vi "d7seg.vi"(0 "Numeric":dbl min=0.0 max=9.0 step=1.0) -> (20 "a":bool, 21 "b":bool, 22 "c":bool, 23 "d":bool, 24 "e":bool, 25 "f":bool, 26 "g":bool, 27 "h":bool)   [LabVIEW 2022 SP3]
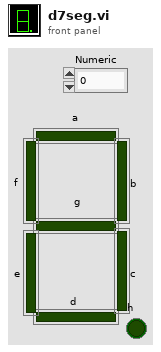
[diagram p1: front panel]
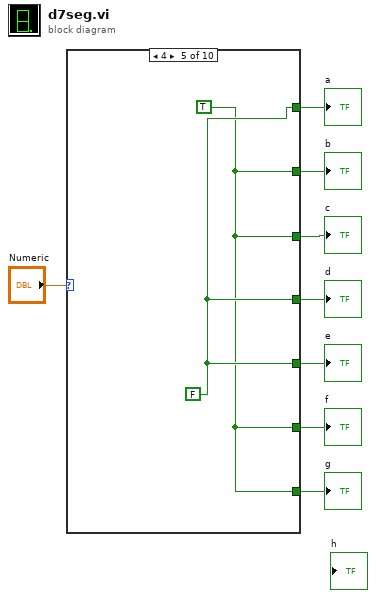
[diagram p0: block diagram]
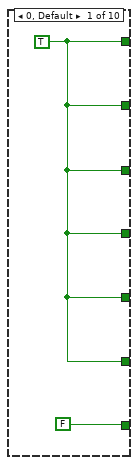
[diagram p2: hidden frame]
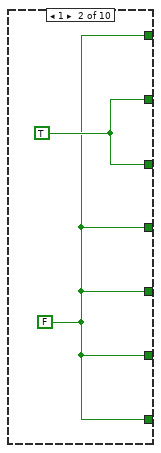
[diagram p3: hidden frame]
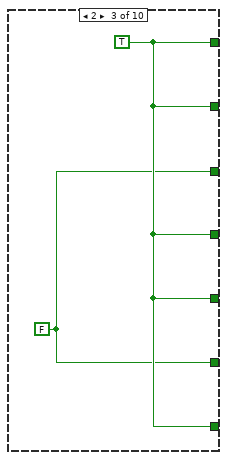
[diagram p4: hidden frame]
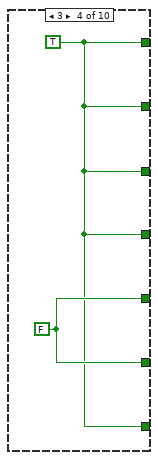
[diagram p5: hidden frame]
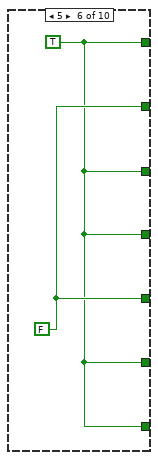
[diagram p6: hidden frame]
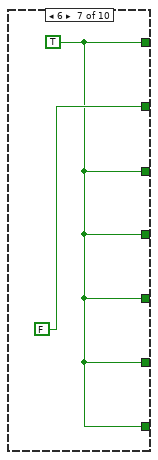
[diagram p7: hidden frame]
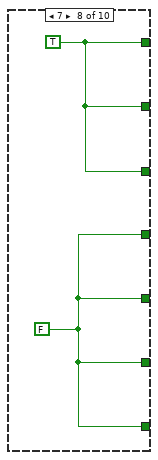
[diagram p8: hidden frame]
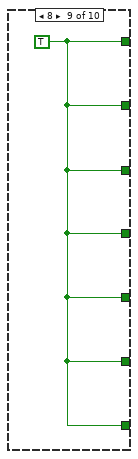
[diagram p9: hidden frame]
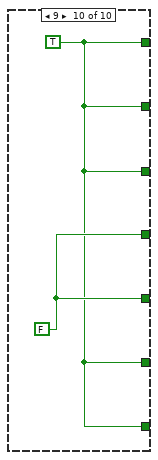
[diagram p10: hidden frame]
diagram:
  n1 = case shown="4" "Numeric" {
    tunnel: [w10 w11 w14 w15 w18 w19 w21 w24 w25 w26] -> w7
    tunnel: [w10 w12 w14 w15 w17 w20 FALSE w24 w25 w26] -> w6
    tunnel: [w10 w12 w13 w15 w17 w19 w21 w24 w25 w26] -> w5
    tunnel: [w10 w11 w14 w15 w18 w19 w21 w23 w25 w27] -> w4
    tunnel: [w10 w11 w14 w16 w18 w20 w21 w23 w25 w27] -> w3
    tunnel: [w10 w11 w13 w16 w17 w19 w21 w23 w25 w26] -> w2
    tunnel: [FALSE w11 w14 w15 w17 w19 w21 w23 w25 w26] -> w1
    frame 0, Default {
      w10 = TRUE
    }
    frame 1 {
      w11 = FALSE
      w12 = TRUE
    }
    frame 2 {
      w13 = FALSE
      w14 = TRUE
    }
    frame 3 {
      w16 = FALSE
      w15 = TRUE
    }
    frame 4 {
      w18 = FALSE
      w17 = TRUE
    }
    frame 5 {
      w20 = FALSE
      w19 = TRUE
    }
    frame 6 {
      w21 = TRUE
    }
    frame 7 {
      w23 = FALSE
      w24 = TRUE
    }
    frame 8 {
      w25 = TRUE
    }
    frame 9 {
      w27 = FALSE
      w26 = TRUE
    }
  }
  "a" <- w7
  "g" <- w1
  "d" <- w4
  "b" <- w6
  "c" <- w5
  "e" <- w3
  "f" <- w2
